vi "Stop.vi"(8 "error in (no error)":errorcluster, 11 "AODAcq in":refnum<class "AODAcq.lvclass">) -> (0 "error out":errorcluster, 3 "AODAcq out":refnum<class "AODAcq.lvclass">)   [LabVIEW 2014, in "AODAcq.lvclass"]
uses:
  AODAcq.lvclass
  <vilib>/Utility/error.llb/Error Cluster From Error Code.vi
  <vilib>/rvi/errors/niLvFpgaAdjustHostInterfaceError.vi
  <vilib>/rvi/interface/nirviMethod/nirviMethod.xnode
  FPGA_Control/AODRef.ctl
  FPGA Bitfiles/AodScanner_FPGATarget_AODControl(FPGA)_TyJc9yYmyGA.lvbitx
  HDF5Tools/LabView/HDF5Tools.lvlib
  <vilib>/rvi/errors/niLvFpgaMergeErrorWithErrorCode.vi
  <vilib>/FPGAPlugInAG/PXIe-7965R/niLvFpga_ReadFifo_PXIe-7965R.vi
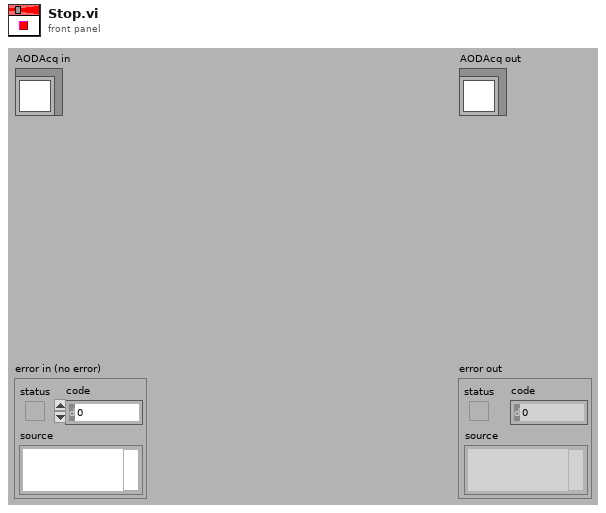
[diagram p1: front panel]
types:
  T1 = cluster{"file handle out":i32, "ImData":i32, "TemporalData":i32, "MotionData":i32, "RawData":i32, "AODMotionCorrectionData":i32, "MotorMotionCorrectionData":i32, "MotionCoordinates":i32, "PointCoordinates":i32}
  T2 = typedef "AODRef.ctl" = refnum<k20>
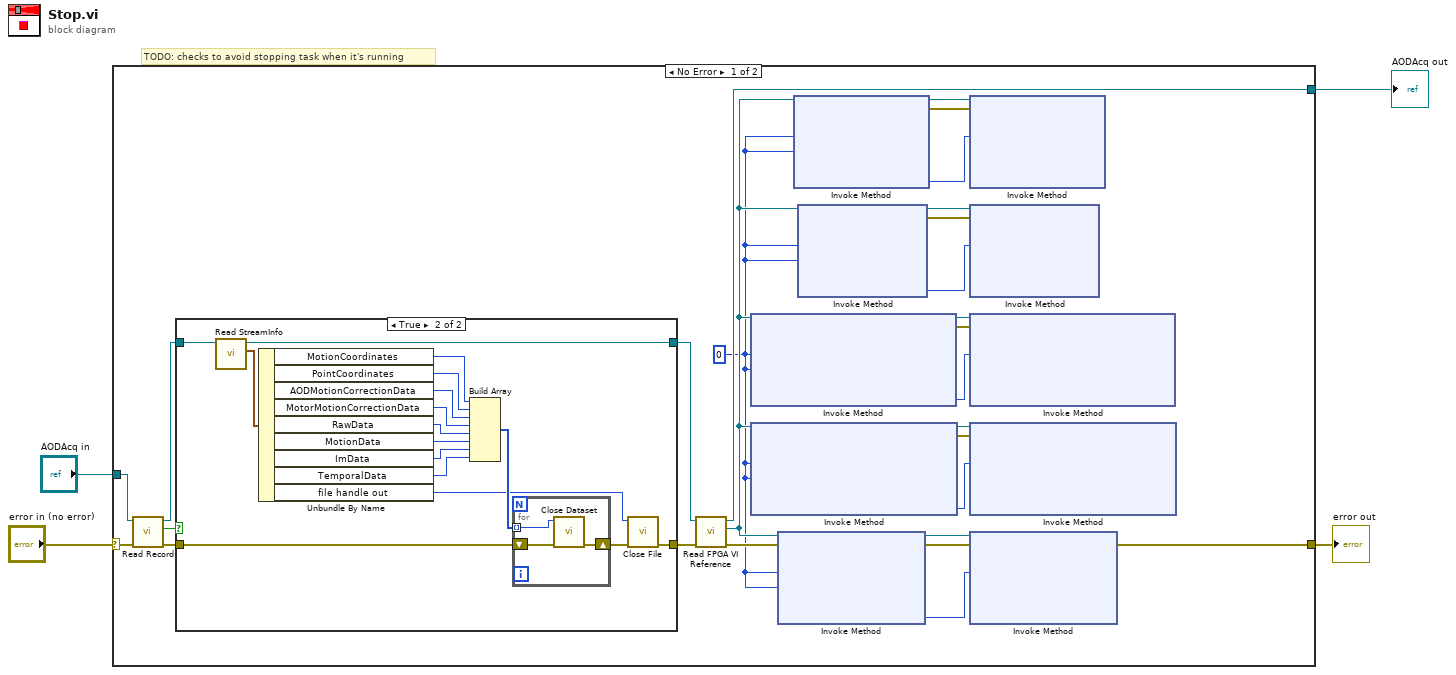
[diagram p0: block diagram]
diagram:
  # "TODO: checks to avoid stopping task when it's running"
  n1 = case shown="No Error" "error in (no error)" {
    selector: "error in (no error)" -> [w19 w54]
    tunnel: [w21 w54] -> w3
    tunnel: [w22 w53] -> w1
    tunnel: "AODAcq in" -> [w18 w53]
    frame No Error {
      w5 = u32 0 ("Number of Elements")
      n2 = call-dynamic "Read Record.vi"("error in (no error)"=w19, "AODAcq in"=w18) -> ("error out"=w15:errorcluster, "Record"=w16:bool, "AODAcq out"=w17:refnum<class "AODAcq.lvclass">)  [unwired: 7 in]
      n3 = case shown="True" w16 {
        tunnel: [w32 w49] -> w20
        tunnel: w17 -> [w32 w38]
        tunnel: w15 -> [w33 w43]
        tunnel: [w33 w40] -> w14
        frame False {
        }
        frame True {
          n4 = call-dynamic "Read StreamInfo.vi"("AODAcq in"=w38) -> ("StreamInfo"=w48:T1, "AODAcq out"=w49:refnum<class "AODAcq.lvclass">)  [unwired: 8 in, 1 out]
          n5 = Unbundle By Name(w48) -> ("MotionCoordinates"=w35:i32, "PointCoordinates"=w34:i32, "AODMotionCorrectionData"=w36:i32, "MotorMotionCorrectionData"=w37:i32, "RawData"=w39:i32, "MotionData"=w45:i32, "ImData"=w46:i32, "TemporalData"=w47:i32, "file handle out"=w42:i32)
          n6 = Build Array(w35, w34, w36, w37, w39, w45, w46, w47) -> (w44:i32[])
          n7 = for {
            tunnel: w44 -> [w52] mode=indexing
            shift-right: [w50] -> w41
            shift-left: w43 -> [w51]
            n8 = call "Close Dataset.vi"("error in (no error)"=w51, "dataset_id"=w52) -> ("error out"=w50:errorcluster)  [unwired: 9 in]
          }
          n9 = call "Close File.vi"("error in (no error)"=w41, "file_id"=w42) -> ("error out"=w40:errorcluster)  [unwired: 9 in]
        }
      }
      n10 = call-dynamic "Read FPGA VI Reference.vi"("error in (no error)"=w14, "AODAcq in"=w20) -> ("error out"=w6:errorcluster, "FPGA VI Reference"=w9:T2, "AODAcq out"=w22:refnum<class "AODAcq.lvclass">)  [unwired: 7 in]
      n11 = xnode "Invoke Method"("FPGA VI Reference In"=w9, "Number of Elements"=w5, "Timeout (ms)"=w5) -> ("FPGA VI Reference Out"=w8:T2, "error out"=w13:errorcluster, "Elements Remaining"=w12:u32)  [unwired: 1 in, 1 out]
      n12 = xnode "Invoke Method"("FPGA VI Reference In"=w9, "Number of Elements"=w5, "Timeout (ms)"=w5) -> ("FPGA VI Reference Out"=w7:T2, "error out"=w11:errorcluster, "Elements Remaining"=w10:u32)  [unwired: 1 in, 1 out]
      n13 = xnode "Invoke Method"("FPGA VI Reference In"=w9, "error in"=w6, "Number of Elements"=w5, "Timeout (ms)"=w5) -> ("FPGA VI Reference Out"=w31:T2, "error out"=w30:errorcluster, "Elements Remaining"=w23:u32)  [unwired: 1 out]
      n14 = xnode "Invoke Method"("FPGA VI Reference In"=w9, "Number of Elements"=w5, "Timeout (ms)"=w5) -> ("FPGA VI Reference Out"=w29:T2, "error out"=w28:errorcluster, "Elements Remaining"=w24:u32)  [unwired: 1 in, 1 out]
      n15 = xnode "Invoke Method"("FPGA VI Reference In"=w9, "Number of Elements"=w5, "Timeout (ms)"=w5) -> ("FPGA VI Reference Out"=w27:T2, "error out"=w26:errorcluster, "Elements Remaining"=w25:u32)  [unwired: 1 in, 1 out]
      n16 = xnode "Invoke Method"("FPGA VI Reference In"=w29, "error in"=w28, "Number of Elements"=w24) -> ()  [unwired: 1 in, 4 out]
      n17 = xnode "Invoke Method"("FPGA VI Reference In"=w27, "error in"=w26, "Number of Elements"=w25) -> ()  [unwired: 1 in, 4 out]
      n18 = xnode "Invoke Method"("FPGA VI Reference In"=w8, "error in"=w13, "Number of Elements"=w12) -> ()  [unwired: 1 in, 4 out]
      n19 = xnode "Invoke Method"("FPGA VI Reference In"=w7, "error in"=w11, "Number of Elements"=w10) -> ()  [unwired: 1 in, 4 out]
      n20 = xnode "Invoke Method"("FPGA VI Reference In"=w31, "error in"=w30, "Number of Elements"=w23) -> ("error out"=w21:errorcluster)  [unwired: 1 in, 3 out]
    }
    frame Error {
    }
  }
  "error out" <- w3
  "AODAcq out" <- w1
